vi "new report subVI.vi"(0 "report in":refnum<class "NI_HTML.lvclass">, 1 "window state (normal)":T1(ring)=enum."normal", 5 "display alerts? (F)":bool, 7 "template (empty)":path, 9 "machine name (empty)":string, 11 "error in (no error)":errorcluster) -> (4 "report out":refnum<class "NI_HTML.lvclass">, 15 "error out":errorcluster)   [LabVIEW 2020, in "NI_HTML.lvclass"]
uses:
  NI_HTML.lvclass
  HTML Report Data.ctl
  NI_HTML.lvclass/NI_HTML.ctl
  NI_ReportGenerationCore.lvlib
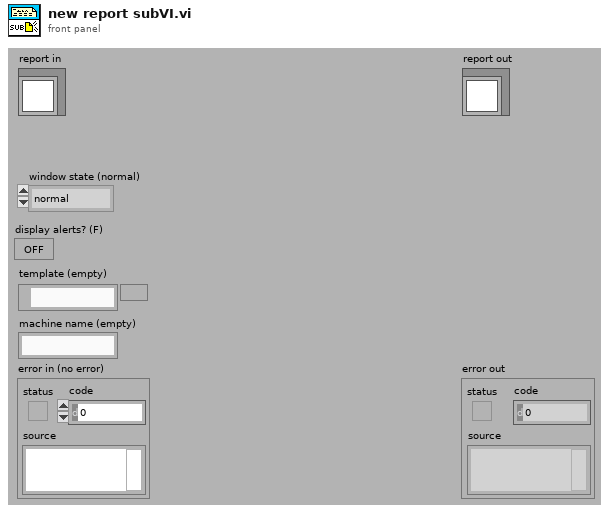
[diagram p1: front panel]
types:
  T1 = enum16{"maximized", "minimized", "normal", "no change"}
  T2 = typedef "NI_ReportGenerationCore.lvlib/HTML Report Data.ctl" = cluster{"Body Text":string, "Font Tag":string, "Title Text":string, "Header Text":string, "Footer Text":string, "Image List":path[]}
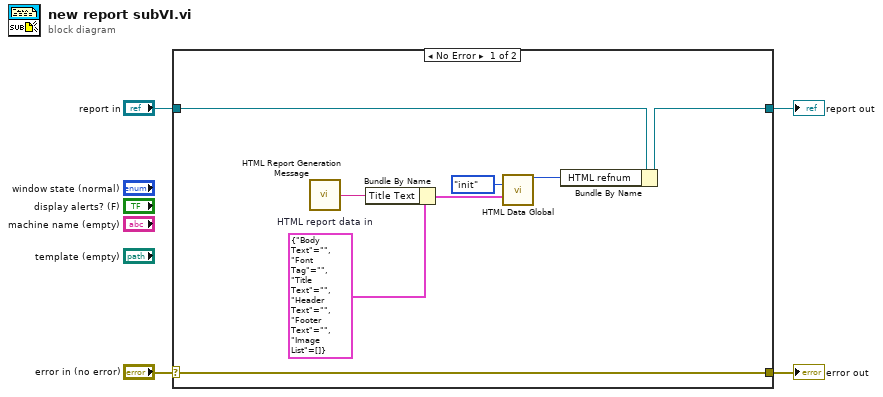
[diagram p0: block diagram]
diagram:
  n1 = case shown="No Error" "error in (no error)" {
    selector: "error in (no error)" -> [w12 w14]
    tunnel: [w12 w14] -> w3
    tunnel: [w10 w13] -> w1
    tunnel: "report in" -> [w11 w13]
    frame No Error {
      w7 = T2 {"Body Text"="", "Font Tag"="", "Title Text"="", "Header Text"="", "Footer Text"="", "Image List"=[]}  # HTML report data in
      n2 = call "HTML Report Generation Message.vi"() -> ("String"=w6:string)
      n3 = Bundle By Name(cluster=w7, "Title Text"=w6) -> (w5:T2)
      n4 = call "HTML Data Global.vi"("menu"=enum16{"init", "get", "set", "delete"}."init", "HTML report data in"=w5) -> ("HTML refnum out"=w9:u32)  [unwired: 1 in, 12 out]
      n5 = Bundle By Name(cluster=w11, "HTML refnum"=w9) -> (w10:refnum<class "NI_HTML.lvclass">)
    }
    frame Error {
    }
  }
  "error out" <- w3
  "report out" <- w1
